vi "改变图片分辨率13版.vi"() -> ()   [LabVIEW 2013]
panel:
  out "new picture":picture caption="原始图片"
  in  "path to BMP file 2":path caption="BMP文件路径"
  out "二维图片":picture
  in  "path to BMP file":path caption="BMP文件路径"
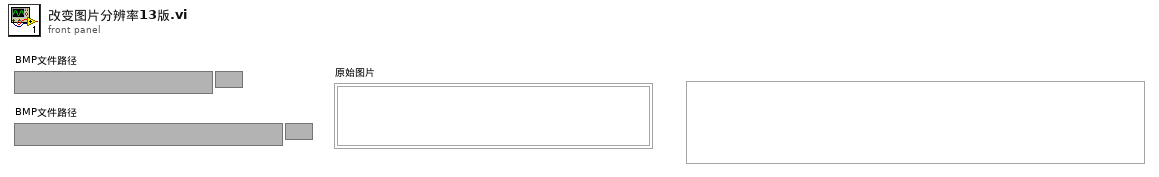
[diagram p1: front panel]
types:
  T1 = typedef "LVBoundsTypeDef.ctl" = cluster{"Width":u32, "Height":u32}
  T2 = typedef "imagedata.ctl" = cluster{"image type":i32, "image depth":i32, "image":u8[], "mask":u8[], "colors":u32[], "Rectangle":cluster{"left":i16, "top":i16, "right":i16, "bottom":i16}}
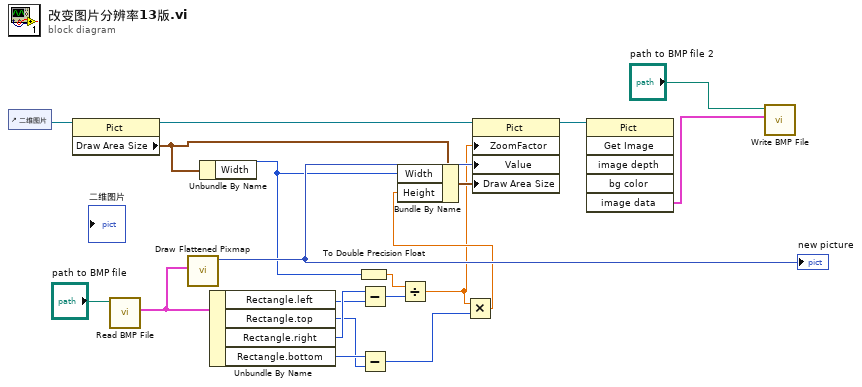
[diagram p0: block diagram]
diagram:
  n1 = control-ref of="二维图片"() -> (w18:refnum<vi>)
  n2 = property class="Pict"(reference=w18) -> (reference out=w17:refnum<vi>, "Draw Area Size"=w2:T1)  [unwired: 1 in, 1 out]
  n3 = call <vilib>:"Read BMP File.vi"("path to BMP file"="path to BMP file") -> ("image data"=w19:T2)  [unwired: 8 in, 2 out]
  n4 = call <vilib>:"Draw Flattened Pixmap.vi"("image data"=w19) -> ("new picture"=w16:picture)  [unwired: 8 in]
  "new picture" <- w16
  n5 = Unbundle By Name(w2) -> ("Width"=w1:u32)
  n6 = Unbundle By Name(w19) -> ("Rectangle.left"=w13:i16, "Rectangle.top"=w11:i16, "Rectangle.right"=w14:i16, "Rectangle.bottom"=w12:i16)
  n7 = To Double Precision Float(number=w1) -> (double precision float=w9:dbl)
  n8 = Subtract(x=w14, y=w13) -> (x-y=w10:i16)
  n9 = Subtract(x=w12, y=w11) -> (x-y=w5:i16)
  n10 = Divide(x=w9, y=w10) -> (x/y=w3:dbl)
  n11 = Multiply(x=w3, y=w5) -> (x*y=w4:dbl)
  n12 = Bundle By Name(cluster=w2, "Width"=w1, "Height"=w4) -> (w15:T1)
  n13 = property class="Pict"(reference=w17, "ZoomFactor"=w3, "Value"=w16, "Draw Area Size"=w15) -> (reference out=w8:refnum<vi>)  [unwired: 1 in, 1 out]
  n14 = invoke class="Pict" method="Get Image"(reference=w8) -> ("image data"=w7:T2)  [unwired: 5 in, 5 out]
  n15 = call <vilib>:"Write BMP File.vi"("image data"=w7, "path to BMP file"="path to BMP file 2") -> ()  [unwired: 8 in, 2 out]
